vi "link.vi"(0 "Attributes":T1, 3 "Name":string="link_name") -> (4 "urdf out":string)   [LabVIEW 2010]
uses:
  LinkAttributes.ctl
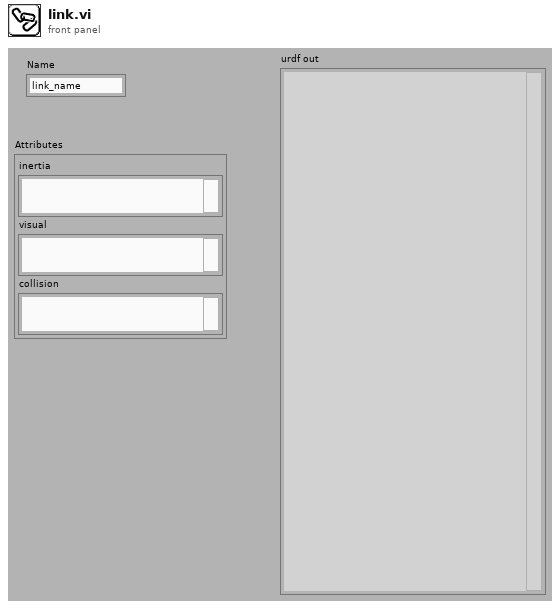
[diagram p1: front panel]
types:
  T1 = typedef "LinkAttributes.ctl" = cluster{"inertia":string, "visual":string, "collision":string}
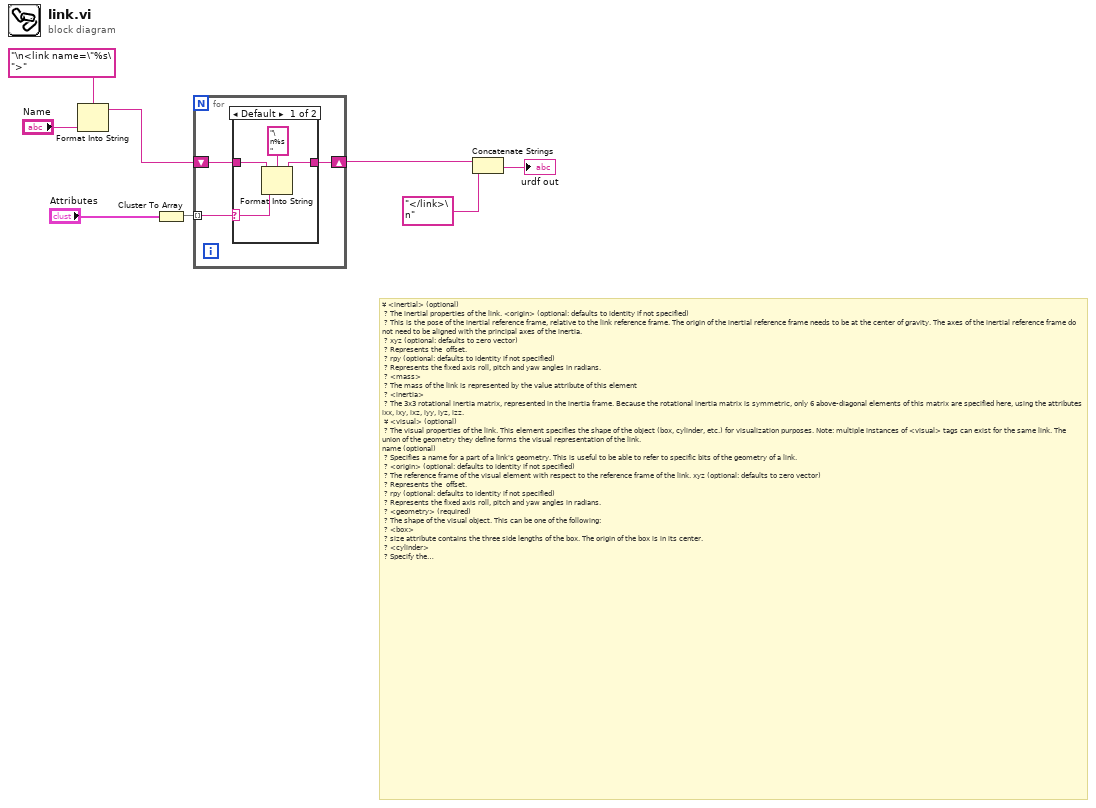
[diagram p0: block diagram]
diagram:
  # "¥\t<inertial> (optional) \n\t?\tThe inertial properties of the link. <origin> (optional: defaults to identity if not specified) \n\t?\tThis is the pose of the inertial reference frame, relative to the link reference frame. The origin of the inertial reference frame needs to be at the center of gravity. The axes of the inertial reference frame do not need to be aligned with the principal axes of the inertia. \n\t?\txyz (optional: defaults to zero vector) \n\t?\tRepresents the  offset. \n\t?\trpy (optional: defaults to identity if not specified) \n\t?\tRepresents the fixed axis roll, pitch and yaw angles in radians.\n\t?\t<mass> \n\t?\tThe mass of the link is represented by the value attribute of this element\n\t?\t<inertia> \n\t?\tThe 3x3 rotational inertia matrix, represented in the inertia frame. Because the rotational inertia matrix is symmetric, only 6 above-diagonal elements of this matrix are specified here, using the attributes ixx, ixy, ixz, iyy, iyz, izz.\n\t¥\t<visual> (optional) \n\t?\tThe visual properties of the link. This element specifies the shape of the object (box, cylinder, etc.) for visualization purposes. Note: multiple instances of <visual> tags can exist for the same link. The union of the geometry they define forms the visual representation of the link. \nname (optional) \n\t?\tSpecifies a name for a part of a link's geometry. This is useful to be able to refer to specific bits of the geometry of a link.\n\t?\t<origin> (optional: defaults to identity if not specified) \n\t?\tThe reference frame of the visual element with respect to the reference frame of the link. xyz (optional: defaults to zero vector) \n\t?\tRepresents the  offset. \n\t?\trpy (optional: defaults to identity if not specified) \n\t?\tRepresents the fixed axis roll, pitch and yaw angles in radians.\n\t?\t<geometry> (required) \n\t?\tThe shape of the visual object. This can be one of the following: \n\t?\t<box> \n\t?\tsize attribute contains the three side lengths of the box. The origin of the box is in its center. \n\t?\t<cylinder> \n\t?\tSpecify the radius and length. The origin of the cylinder is in its center. \n\t?\t<sphere> \n\t?\tSpecify the radius. The origin of the sphere is in its center. \n\t?\t<mesh> \n\t?\tA trimesh element specified by a filename, and an optional scale that scales the mesh's axis-aligned-bounding-box. The recommended format for best texture and color support is Collada .dae files, though .stl files are also supported. The mesh file is not transferred between machines referencing the same model. It must be a local file. \n\t?\t<material> (optional) \n\t?\tThe material of the visual element. It is allowed to specify a material element outside of the 'link' object, in the top level 'robot' element. From within a link element you can then reference the material by name.\n\t?\tname name of the material \n\t?\t<color> (optional) \n\t?\trgba The color of a material specified by set of four numbers representing red/green/blue/alpha, each in the range of [0,1]. \n\t?\t<texture> (optional) \n\t?\tThe texture of a material is specified by a filename \n\t¥\t<collision> (optional) \n\t?\tThe collision properties of a link. Note that this can be different from the visual properties of a link, for example, simpler collision models are often used to reduce computation time. Note: multiple instances of <collision> tags can exist for the same link. The union of the geometry they define forms the collision representation of the link. \nname (optional) \n\t?\tSpecifies a name for a part of a link's geometry. This is useful to be able to refer to specific bits of the geometry of a link.\n\t?\t<origin> (optional: defaults to identity if not specified) \n\t?\tThe reference frame of the collision element, relative to the reference frame of the link. xyz (optional: defaults to zero vector) \n\t?\tRepresents the  offset. \n\t?\trpy (optional: defaults to identity if not specified) \n\t?\tRepresents the fixed axis roll, pitch and yaw angles in radians.\n\t?\t<geometry> \n\t?\tSee the geometry description in the above visual element."
  n1 = Format Into String(format string="\n<link name=\"%s\">", "Name") -> (resulting string=w8:string)  [unwired: 2 in, 1 out]
  n2 = Cluster To Array(cluster="Attributes") -> (array=w1:string[])
  n3 = for {
    shift-right: [w11] -> w5
    shift-left: w8 -> [w10]
    tunnel: w1 -> [w9] mode=indexing
    n4 = case shown="Default" w9 {
      selector: w9 -> [w13 _]
      tunnel: [w12 w16] -> w11
      tunnel: w10 -> [w15 w16]
      frame Default {
        n5 = Format Into String(format string="\n%s", initial string=w15, w13) -> (resulting string=w12:string)  [unwired: 1 in, 1 out]
      }
      frame "" {
      }
    }
  }
  n6 = Concatenate Strings(w5, "</link>\n") -> (→"urdf out":string)
